vi "JSON Unflatten Configuration.vi"(8 "error in (no error)":errorcluster, 10 "dsf version":T13, 11 "dsf configuration json":string) -> (0 "error out":errorcluster, 3 "framework configuration":T1)   [LabVIEW 2017, in "DSF Core.lvlib" / "Configuration Session.lvclass"]
uses:
  Configuration Session.lvclass
  Typedefs/DSF Version Info.ctl
  Typedefs/DSF Engine Framework Configuration.ctl
  Typedefs/DSF Engine Plugin Configuration.ctl
  Typedefs/DSF Timing Info.ctl
  Typedefs/DSF Engine Plugin Thread Configuration.ctl
  Typedefs/DSF Settings Info.ctl
  Typedefs/DSF Engine Transfer Group Configuration.ctl
  Typedefs/DSF Direction.ctl
  Typedefs/DSF Engine Transfer Configuration.ctl
  Typedefs/DSF Byte Order.ctl
  Typedefs/DSF Engine Channel Configuration.ctl
  Typedefs/DSF Data Type.ctl
  Typedefs/DSF Timeout Behavior.ctl
  DSF Core.lvlib
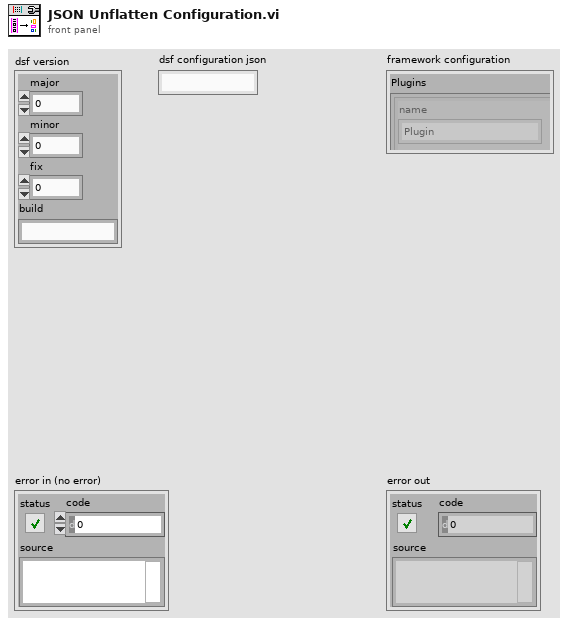
[diagram p1: front panel]
types:
  T1 = typedef "DSF Core.lvlib/DSF Engine Framework Configuration.ctl" = cluster{"Plugins":T2[]}
  T2 = typedef "DSF Core.lvlib/DSF Engine Plugin Configuration.ctl" = cluster{"name":string, "components":string[], "cycle timing":T3, "threads":T4[], "Transfer Groups":T6[], "settings":T5}
  T3 = typedef "DSF Core.lvlib/DSF Timing Info.ctl" = cluster{"priority":u64, "decimation":u64, "offset":u64}
  T4 = typedef "DSF Core.lvlib/DSF Engine Plugin Thread Configuration.ctl" = cluster{"buffer converter settings":T5, "transceiver settings":T5, "custom settings":T5, "processor":i32, "priority offset":i16}
  T5 = typedef "DSF Core.lvlib/DSF Settings Info.ctl" = cluster{"key":string, "value":string}[]
  T6 = typedef "DSF Core.lvlib/DSF Engine Transfer Group Configuration.ctl" = cluster{"name":string, "direction":T7, "cycle timing":T3, "thread index":i32, "settings":T5, "Transfers":T8[], "timeout behavior":T12}
  T7 = typedef "DSF Core.lvlib/DSF Direction.ctl" = enum8{"Tx", "Rx"}
  T8 = typedef "DSF Core.lvlib/DSF Engine Transfer Configuration.ctl" = cluster{"name":string, "byte order":T9, "settings":T5, "channels":T10[]}
  T9 = typedef "DSF Core.lvlib/DSF Byte Order.ctl" = enum8{"big-endian", "little-endian"}
  T10 = typedef "DSF Core.lvlib/DSF Engine Channel Configuration.ctl" = cluster{"string offset":u64, "string data type":T11, "engine data type":T11, "name":string, "settings":T5, "units":string}
  T11 = typedef "DSF Core.lvlib/DSF Data Type.ctl" = enum8{"Bool", "SGL", "DBL", "I8", "I16", "I32", "I64", "U8", "U16", "U32", "U64"}
  T12 = typedef "DSF Core.lvlib/DSF Timeout Behavior.ctl" = enum8{"Increment Late Count", "Throw Error"}
  T13 = typedef "DSF Core.lvlib/DSF Version Info.ctl" = cluster{"major":u32, "minor":u32, "fix":u32, "build":string}
  T14 = typedef "DSF Core.lvlib/Configuration Session.lvclass/Configuration 1.1.ctl" = cluster{"Plugins":cluster{"name":string, "components":string[], "cycle timing":cluster{"priority":u64, "decimation":u64, "offset":u64}, "threads":cluster{"buffer converter settings":cluster{"key":string, "value":string}[], "transceiver settings":cluster{"key":string, "value":string}[], "custom settings":cluster{"key":string, "value":string}[], "processor":i32, "priority offset":i16}[], "Transfer Groups":cluster{"name":string, "direction":enum8{"Tx", "Rx"}, "cycle timing":cluster{"priority":u64, "decimation":u64, "offset":u64}, "thread index":i32, "settings":cluster{"key":string, "value":string}[], "Transfers":cluster{"name":string, "byte order":enum8{"big-endian", "little-endian"}, "settings":cluster{"key":string, "value":string}[], "channels":cluster{"string offset":u64, "string data type":enum8{"Bool", "SGL", "DBL", "I8", "I16", "I32", "I64", "U8", "U16", "U32", "U64"}, "engine data type":enum8{"Bool", "SGL", "DBL", "I8", "I16", "I32", "I64", "U8", "U16", "U32", "U64"}, "name":string, "settings":cluster{"key":string, "value":string}[], "units":string}[]}[], "timeout behavior":enum8{"Increment Late Count", "Throw Error"}}[], "settings":cluster{"key":string, "value":string}[]}[]}
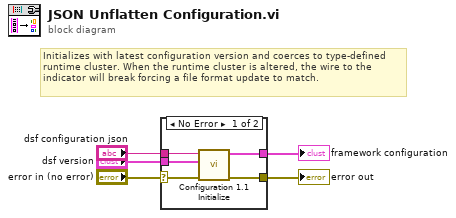
[diagram p0: block diagram]
diagram:
  # "Initializes with latest configuration version and coerces to type-defined runtime cluster. When the runtime cluster is altered, the wire to the indicator will break forcing a file format update to match."
  n1 = case shown="No Error" "error in (no error)" {
    selector: "error in (no error)" -> [w6 w11]
    tunnel: [w10 w11] -> w5
    tunnel: "dsf configuration json" -> [w9 _]
    tunnel: "dsf version" -> [w8 _]
    tunnel: [w7 _] -> w2
    frame No Error {
      n2 = call "Configuration 1.1 Initialize.vi"("error in (no error)"=w6, "dsf version"=w8, "dsf configuration json"=w9) -> ("error out"=w10:errorcluster, "framework configuration 1.1"=w7:T14)  [unwired: 7 in]
    }
    frame Error {
    }
  }
  "error out" <- w5
  "framework configuration" <- w2
